vi "Configure Microwave Input.vi"(8 "error in (no error)":errorcluster, 9 "Center Frequency (300 MHz)":dbl=300000000.0, 10 "Acquisition (T: On)":bool=TRUE, 11 "VISA resource name":refnum<visa-resource-name>) -> (0 "error out":errorcluster, 3 "VISA resource name out":refnum<visa-resource-name>)   [LabVIEW 2019, in "Pendulum CNT90.lvlib"]
doc: "Switches the automatic acquisition system On or Off and sets the center frequency value for the RF input. Center frequency is used when Manual Acquisition has been selected.\n\n<B>Note:</B> VI is intended for use with CNT-90XL only."
uses:
  Pendulum CNT90.lvlib
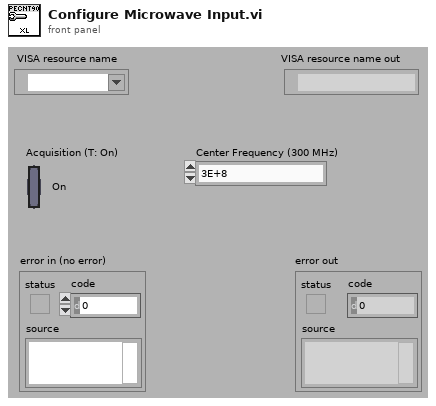
[diagram p1: front panel]
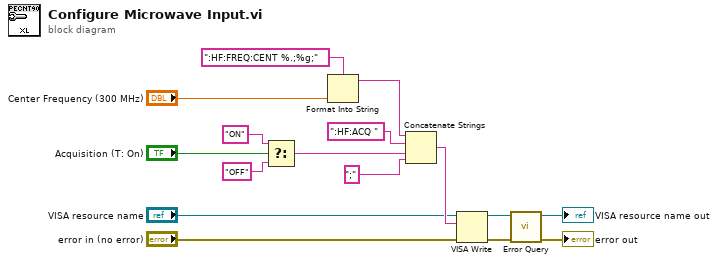
[diagram p0: block diagram]
diagram:
  n1 = Select(t="ON", s="Acquisition (T: On)", f="OFF") -> (s? t:f=w12:string)
  n2 = Format Into String(format string=":HF:FREQ:CENT %.;%g;" ("Attenuation Command"), "Center Frequency (300 MHz)") -> (resulting string=w14:string)  [unwired: 2 in, 1 out]
  n3 = Concatenate Strings(w14, ":HF:ACQ ", w12, ";") -> (w10:string)
  n4 = VISA Write(VISA resource name="VISA resource name", write buffer=w10, error in (no error)="error in (no error)") -> (VISA resource name out=w3:refnum<visa-resource-name>, error out=w4:errorcluster)  [unwired: 1 out]
  n5 = call "Error Query.vi"("error in (no error)"=w4, "VISA resource name"=w3) -> ("error out"=→"error out":errorcluster, "VISA resource name out"=→"VISA resource name out":refnum<visa-resource-name>)  [unwired: 6 in, 2 out]
